vi "Revision Query.vi"(8 "Error in (no error)":errorcluster, 10 "THM1176 Description":string, 11 "VISA resource":refnum<visa-resource-name>) -> (0 "Error out":errorcluster, 1 "Instrument Driver Revision":string, 2 "Info":string, 3 "Dup VISA resource":refnum<visa-resource-name>, 4 "Cal Date":string, 5 "Cal > 18 mo?":bool, 6 "F/W version":dbl)   [LabVIEW 2010]
doc: "Copyright (c) 2012 Metrolab Technology SA, Plan-les-Ouates, Geneva, Switzerland\nQueries the current instrument firmware revision and instrument driver revision."
uses:
  <vilib>/Utility/miscctls.llb/LVDateTimeRec.ctl
panel:
  in  "date time rec":T1
  # "Revision Query"
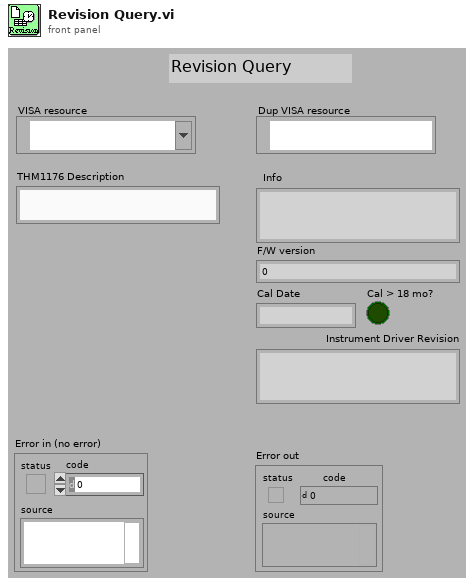
[diagram p1: front panel]
types:
  T1 = typedef "LVDateTimeRec.ctl" = cluster{"fractional second":dbl, "second":i32, "minute":i32, "hour":i32, "day of month":i32, "month":i32, "year":i32, "day of week":i32, "day of year":i32, "DST":i32}
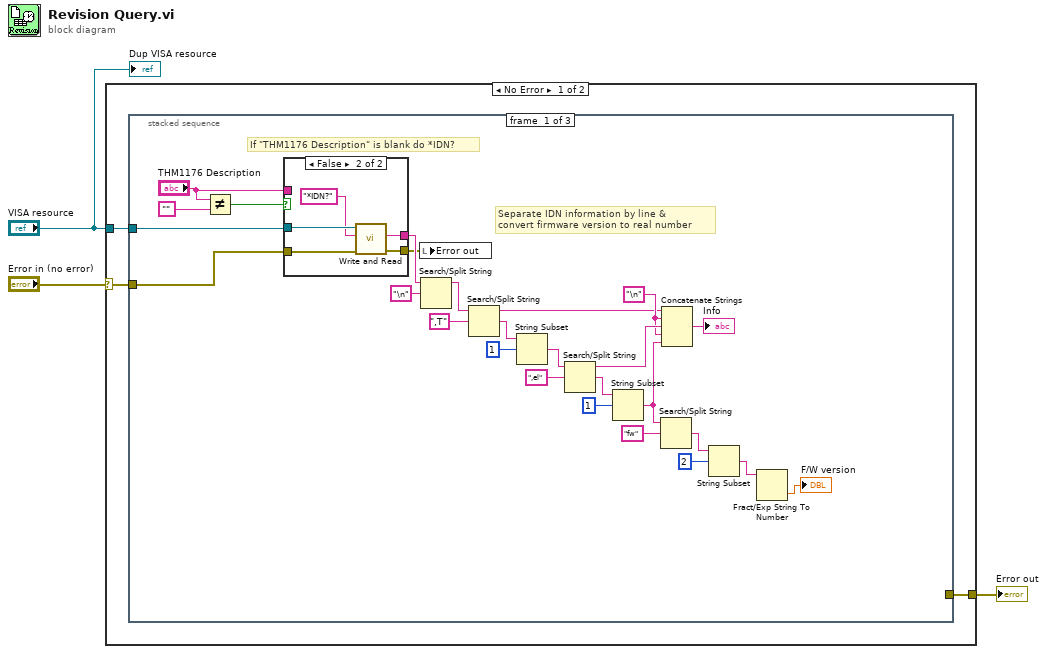
[diagram p0: block diagram]
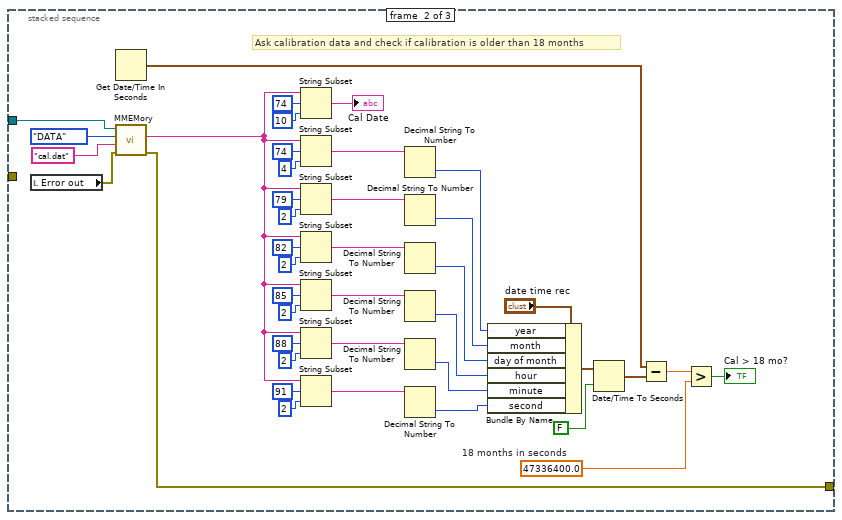
[diagram p3: hidden frame]
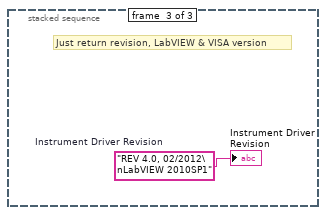
[diagram p4: hidden frame]
diagram:
  n1 = case shown="No Error" "Error in (no error)" {
    selector: "Error in (no error)" -> [w4 w82]
    tunnel: "VISA resource" -> [w6 _]
    tunnel: [w5 w82] -> w3
    frame No Error {
      n2 = stacked-sequence {
        tunnel: w6 -> [w11 w76 _]
        tunnel: [_ w42 _] -> w5
        tunnel: w4 -> [w10 _ _]
        frame #0 {
          w21 = "\n" ("string")
          # "Separate IDN information by line & \nconvert firmware version to real number"
          # "If \"THM1176 Description\" is blank do *IDN?"
          n3 = Not Equal?(x="THM1176 Description", y="") -> (x != y?=w12:bool)
          n4 = case shown="False" w12 {
            tunnel: [w34 w36] -> w7
            tunnel: w11 -> [_ w39]
            tunnel: w10 -> [w34 w38]
            tunnel: [w33 w35] -> w8
            tunnel: "THM1176 Description" -> [w33 _]
            frame True {
            }
            frame False {
              n5 = call "Write and Read.vi"("Error in (no error)"=w38, "Command"="*IDN?", "VISA resource"=w39) -> ("Error out"=w36:errorcluster, "Response"=w35:string)  [unwired: 4 in, 3 out]
            }
          }
          n6 = local write "Error out"(w7) -> ()
          n7 = Search/Split String(string=w8, search string/char (-)="\n") -> (substring before match=w16:string)  [unwired: 1 in, 2 out]
          n8 = Search/Split String(string=w16, search string/char (-)=",T") -> (substring before match=w18:string, match + rest of string=w20:string)  [unwired: 1 in, 1 out]
          n9 = String Subset(string=w20, offset (0)=1) -> (substring=w23:string)  [unwired: 1 in]
          n10 = Search/Split String(string=w23, search string/char (-)=",el") -> (substring before match=w24:string, match + rest of string=w26:string)  [unwired: 1 in, 1 out]
          n11 = String Subset(string=w26, offset (0)=1) -> (substring=w28:string)  [unwired: 1 in]
          n12 = Search/Split String(string=w28, search string/char (-)="fw") -> (match + rest of string=w30:string)  [unwired: 1 in, 2 out]
          n13 = Concatenate Strings(w18, w21, w24, w21, w28) -> (→"Info":string)
          n14 = String Subset(string=w30, offset (0)=2) -> (substring=w31:string)  [unwired: 1 in]
          n15 = Fract/Exp String To Number(string=w31) -> (number=→"F/W version":dbl)  [unwired: 3 in, 1 out]
        }
        frame #1 {
          w45 = 47336400.0  # 18 months in seconds
          # "Ask calibration data and check if calibration is older than 18 months"
          n16 = local read "Error out"() -> (w40:errorcluster)
          n17 = Get Date/Time In Seconds() -> (seconds since 1Jan1904=w47:timestamp)
          n18 = call "MMEMory.vi"("Error in (no error)"=w40, "Filename"="cal.dat", "What"=enum16{"CATalog", "DATA"}."DATA", "VISA resource"=w76) -> ("Error out"=w42:errorcluster, "Response"=w60:string)  [unwired: 5 in, 1 out]
          n19 = String Subset(string=w60, offset (0)=74, length (rest)=10 ("length (rest)")) -> (substring=→"Cal Date":string)
          n20 = String Subset(string=w60, offset (0)=74, length (rest)=4 ("length (rest)")) -> (substring=w69:string)
          n21 = String Subset(string=w60, offset (0)=79, length (rest)=2 ("length (rest)")) -> (substring=w68:string)
          n22 = String Subset(string=w60, offset (0)=82, length (rest)=2 ("length (rest)")) -> (substring=w67:string)
          n23 = String Subset(string=w60, offset (0)=85, length (rest)=2 ("length (rest)")) -> (substring=w59:string)
          n24 = String Subset(string=w60, offset (0)=88, length (rest)=2 ("length (rest)")) -> (substring=w58:string)
          n25 = String Subset(string=w60, offset (0)=91, length (rest)=2 ("length (rest)")) -> (substring=w57:string)
          n26 = Decimal String To Number(string=w69) -> (number=w51:i32)  [unwired: 2 in, 1 out]
          n27 = Decimal String To Number(string=w68) -> (number=w52:i32)  [unwired: 2 in, 1 out]
          n28 = Decimal String To Number(string=w67) -> (number=w53:i32)  [unwired: 2 in, 1 out]
          n29 = Decimal String To Number(string=w59) -> (number=w54:i32)  [unwired: 2 in, 1 out]
          n30 = Decimal String To Number(string=w58) -> (number=w55:i32)  [unwired: 2 in, 1 out]
          n31 = Decimal String To Number(string=w57) -> (number=w56:i32)  [unwired: 2 in, 1 out]
          n32 = Bundle By Name(cluster="date time rec", "year"=w51, "month"=w52, "day of month"=w53, "hour"=w54, "minute"=w55, "second"=w56) -> (w50:T1)
          n33 = Date/Time To Seconds(1:FALSE ("to UTC (F)"), 2:w50) -> (0:w48:timestamp)
          n34 = Subtract(x=w47, y=w48) -> (x-y=w46:dbl)
          n35 = Greater?(x=w46, y=w45) -> (0:→"Cal > 18 mo?":bool)
        }
        frame #2 {
          w81 = "REV 4.0, 02/2012\nLabVIEW 2010SP1"  # Instrument Driver Revision
          # "Just return revision, LabVIEW & VISA version"
          "Instrument Driver Revision" <- w81
        }
      }
    }
    frame Error {
    }
  }
  "Error out" <- w3
  "Dup VISA resource" <- "VISA resource"
